vi "总氮总磷质控流程.vi"(0 "队列输入TP":refnum<queue>, 5 "总氮量程切换":enum32{"H", "L", "AUTO"}(ring)=enum."AUTO", 7 "总磷量程切换":enum32{"H", "L", "AUTO"}(ring)=enum."AUTO", 9 "总磷":bool, 11 "总氮":bool) -> (4 "布尔":bool, 6 "总磷中断报警":bool, 8 "总氮中断报警":bool)   [LabVIEW 2016, in "质控单元.lvlib"]
panel:
  out "总磷":bool
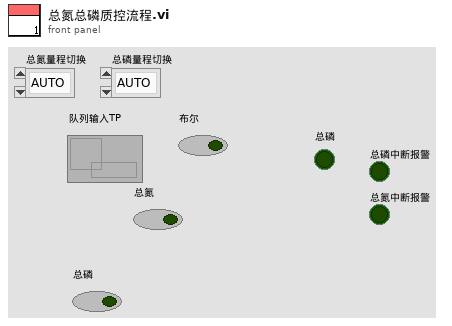
[diagram p1: front panel]
types:
  T1 = enum16{"待机", "启动氨氮水样", "氨氮测量中", "启动氨氮加标", "启动氨氮加标回收", "氨氮加标回收测量中", "启动总氮水样", "总氮测量中", "启动总氮加标", "启动总氮加标回收", "总氮加标回收测量中", "启动总磷水样", "总磷水样测量中", "启动总磷加标", "启动总磷加标回收", "总磷加标回收测量中", "结束"}
  T2 = cluster{"站号":u16, "量程切换":enum32{"H", "L", "AUTO"}, "控制命令":enum16{"启动测量", "标样核查", "零点核查", "跨度核查", "空白测试", "平行样测试", "加标回收", "空白校准", "标样校准", "初始化（清洗）", "停止测试", "仪器重启", "校时", "模式设置", "测量间隔设置"}, "模式设置":enum16{"待机", "连续模式", "周期模式", "定点模式", "受控模式", "手动模式"}, "测量间隔":u16}
  T3 = cluster{"时间标识":timestamp, "设备":string, "日志信息":string}
  T4 = cluster{"系统时间":timestamp, "工作状态":enum16{"空闲", "水样测试", "标样核查", "零点核查", "跨度核查", "空白测试", "平行样测试", "加标回收", "空白校准", "标样校准", "初始化（清洗）"}, "测量模式":enum16{"待机", "连续模式", "周期模式", "定点模式", "受控模式", "手动模式"}, "告警代码":enum16{"无告警", "缺试剂告警", "缺水样告警", "缺蒸馏水告警", "缺标液告警", "仪表漏液告警", "标定异常告警", "超量程告警", "加热异常", "低试剂预警", "超上限告警", "超下限告警", "仪表内部其他异常", "滴定异常告警", "电极异常告警", "量程切换告警", "参数设置告警", "PH电极电位异常", "电导率电极异常", "浊度光度异常", "溶解氧电极异常", "溶解氧光强异常", "温度异常告警", "PH异常告警", "溶解氧异常告警", "电导率异常告警", "浊度异常告警", "叶绿素异常告警", "藻密度异常告警", "蓝绿藻异常告警", "ORP异常告警", "氨氮异常告警", "清洁刷异常告警", "SD卡异常告警", "蓝牙异常告警", "Wifi异常告警", "流程异常告警"}, "故障代码":enum16{"无故障", "电机故障", "温度故障", "通讯故障", "滴定故障"}, "日志代码":u16, "软件版本":u16, "F0":sgl, "F1":sgl, "F2":sgl, "F3":sgl, "T":sgl, "H":sgl, "id":u16, "flowid":u16, "量程":u16, "总磷控温温度1":sgl, "营养盐控温温度2":sgl, "ADC":sgl}
  T5 = enum16{"空闲", "水样测试", "标样核查", "零点核查", "跨度核查", "空白测试", "平行样测试", "加标回收", "空白校准", "标样校准", "初始化（清洗）"}
  T6 = cluster{"因子编码":u32, "单位":u16, "标样参考值":sgl, "水样数据时间":timestamp, "水样实测值":sgl, "水样数据标识":string, "标样数据时间":timestamp, "标样实测值":sgl, "标样数据标识":string, "空白数据时间":timestamp, "空白实测值":sgl, "空白数据标识":string, "零点核查数据时间":timestamp, "零点核查实测值":sgl, "零点核查数据标识":string, "跨度核查数据时间":timestamp, "跨度核查实测值":sgl, "跨度核查数据标识":string, "加标回收数据时间":timestamp, "加标回收实测值":sgl, "加标回收数据标识":string, "平行样数据时间":timestamp, "平行样实测值":sgl, "平行样数据标识":string}
  T7 = cluster{"量程":dbl, "检出限":dbl, "加标前水样浓度":dbl, "加标后水样浓度":dbl, "加标水杯定容体积":dbl, "加标母液浓度":dbl, "加标体积":dbl, "加标回收率":dbl}
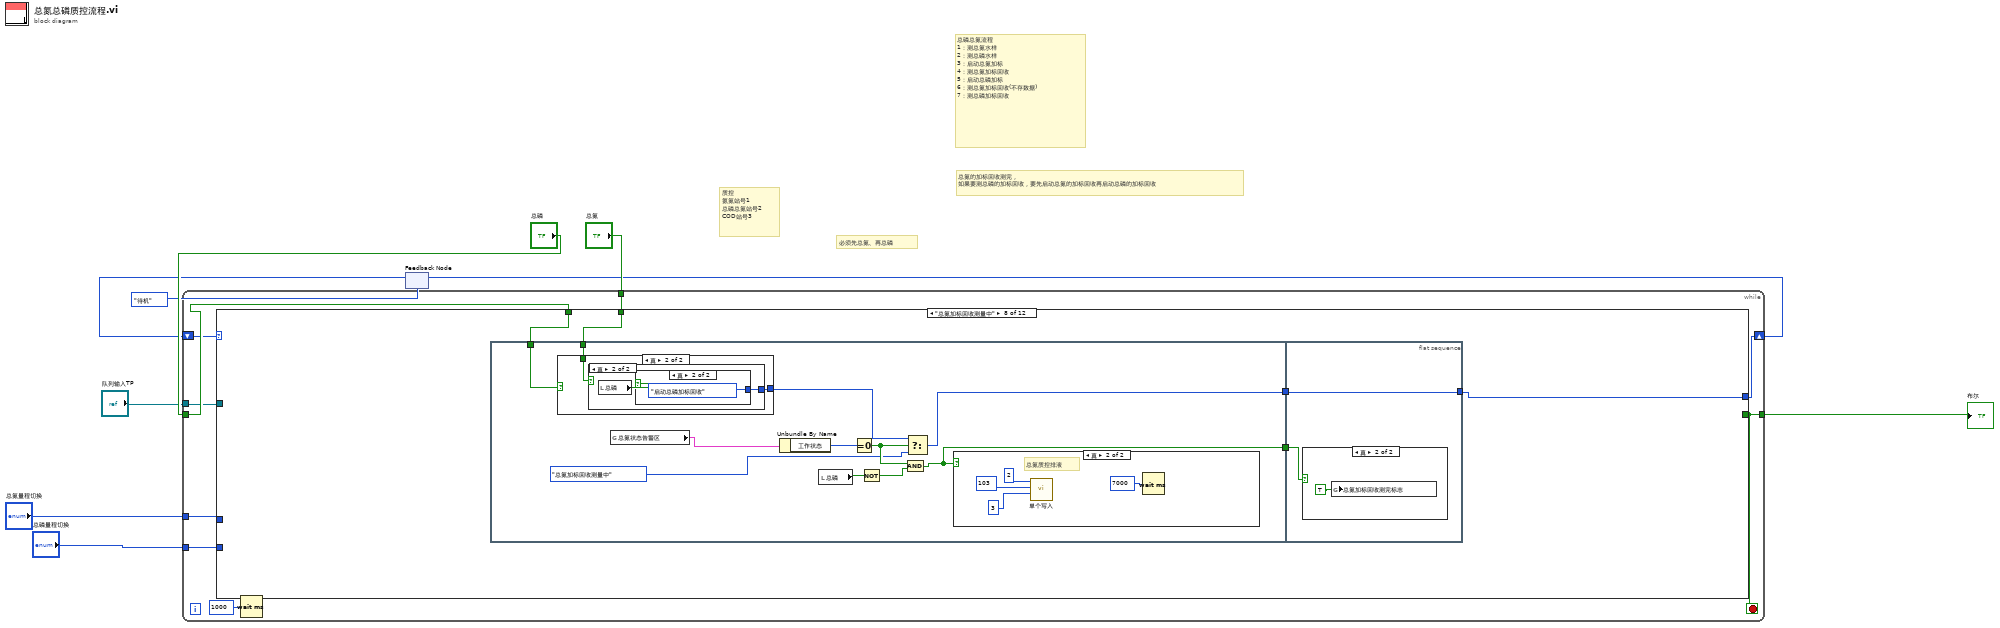
[diagram p0: block diagram]
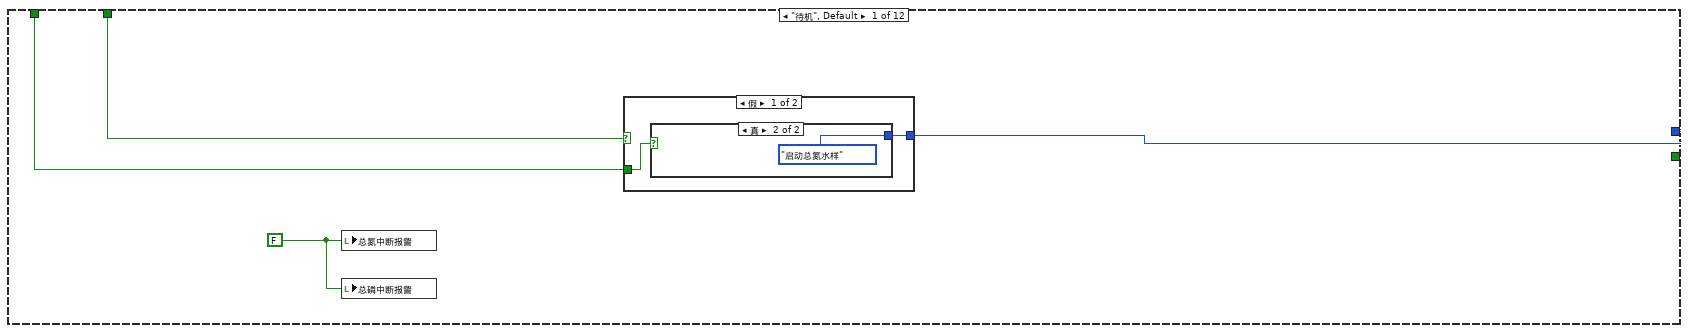
[diagram p2: hidden frame]
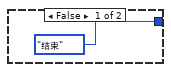
[diagram p3: hidden frame]
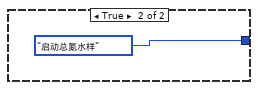
[diagram p4: hidden frame]
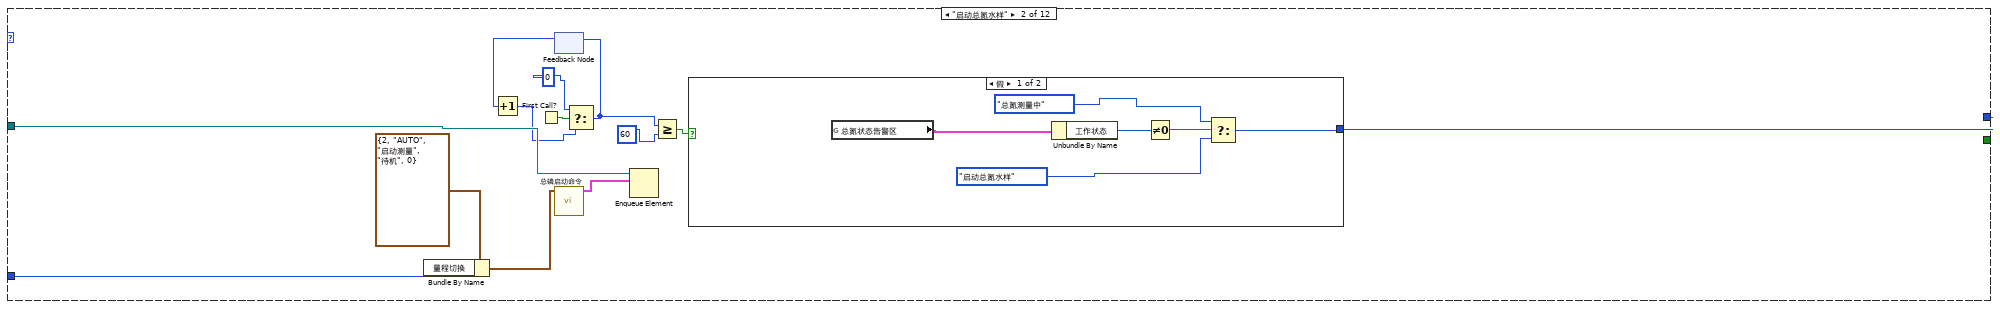
[diagram p5: hidden frame]
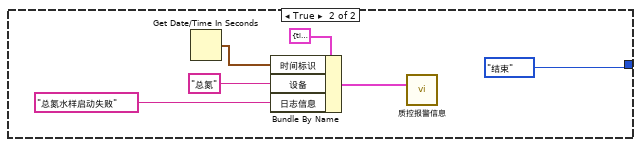
[diagram p6: hidden frame]
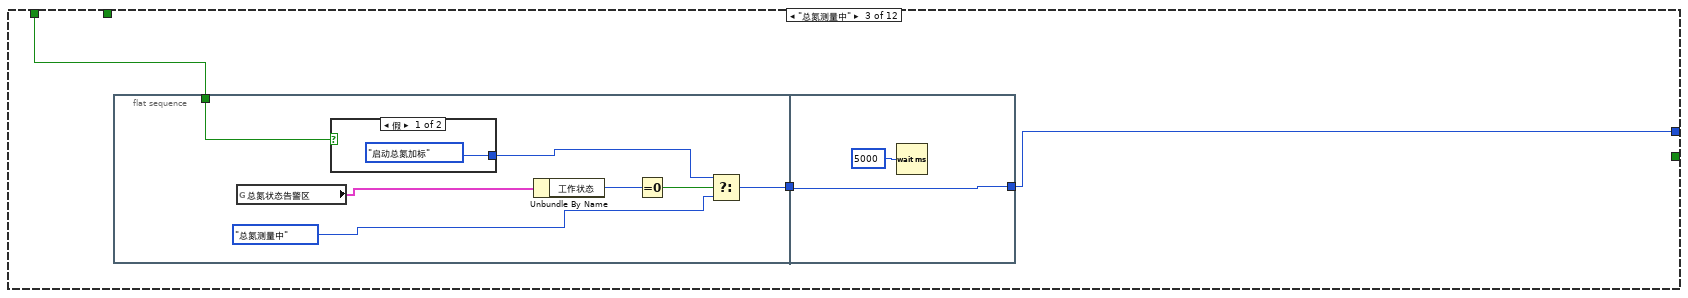
[diagram p7: hidden frame]
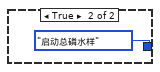
[diagram p8: hidden frame]
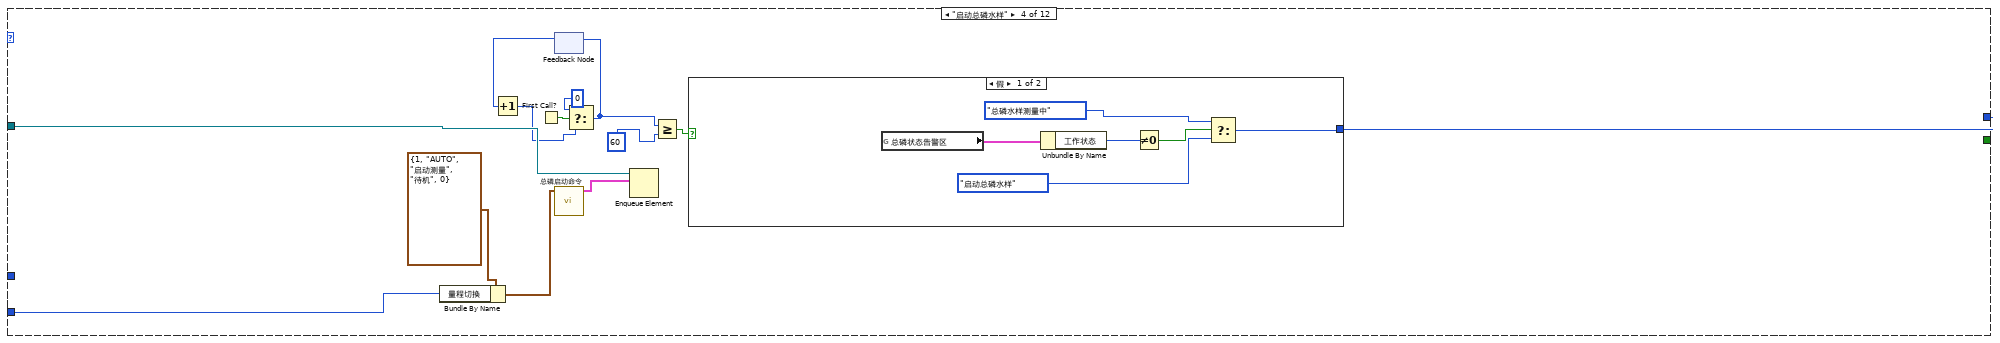
[diagram p9: hidden frame]
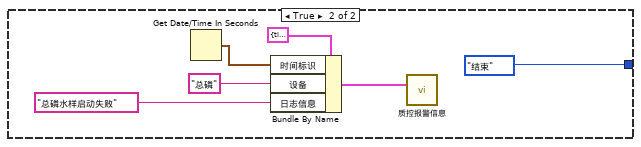
[diagram p10: hidden frame]
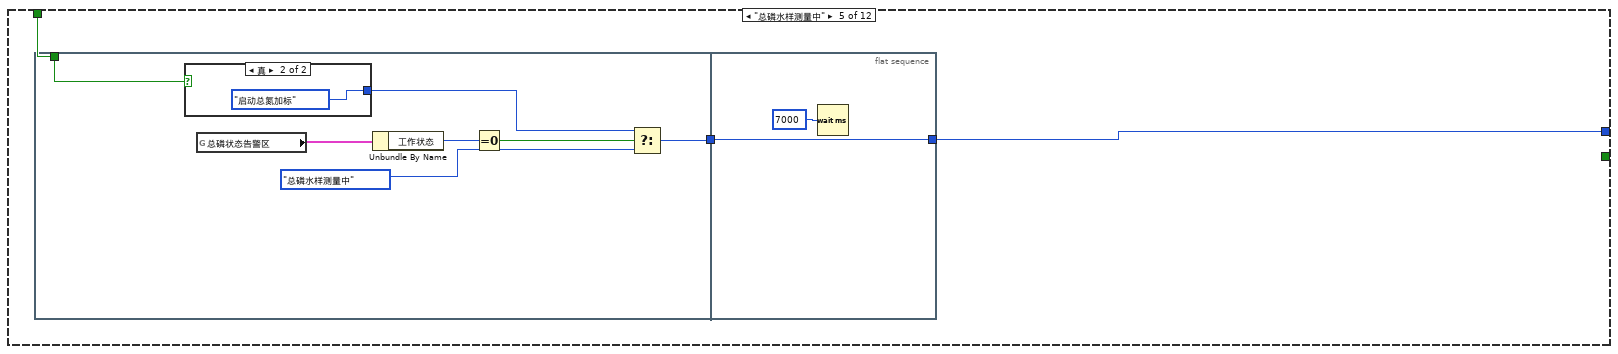
[diagram p11: hidden frame]
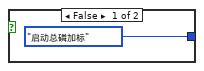
[diagram p12: hidden frame]
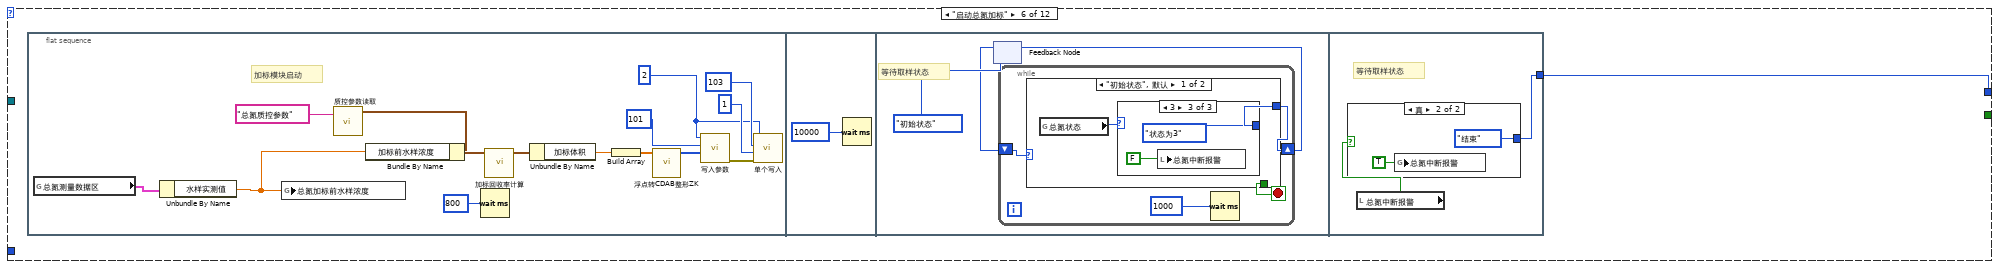
[diagram p13: hidden frame]
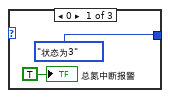
[diagram p14: hidden frame]
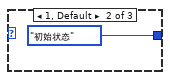
[diagram p15: hidden frame]
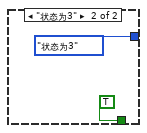
[diagram p16: hidden frame]
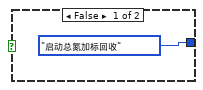
[diagram p17: hidden frame]
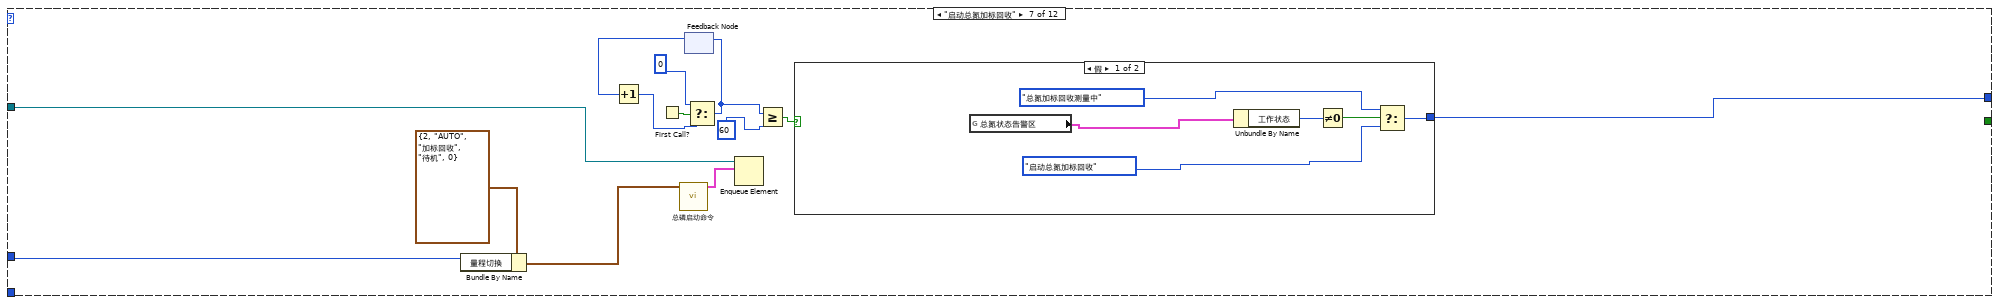
[diagram p18: hidden frame]
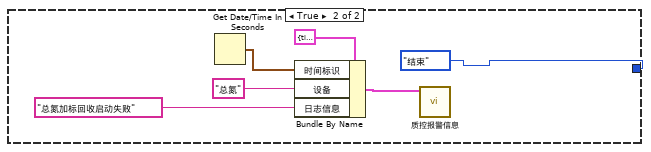
[diagram p19: hidden frame]
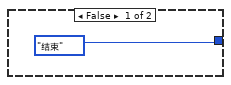
[diagram p20: hidden frame]
diagram:
  # "总磷总氮流程\n1：测总氮水样\n2：测总磷水样\n3：启动总氮加标\n4：测总氮加标回收\n5：启动总磷加标\n6：测总氮加标回收(不存数据)\n7：测总磷加标回收"
  # "总氮的加标回收测完，\n如果要测总磷的加标回收，要先启动总氮的加标回收再启动总磷的加标回收"
  # "质控\n氨氮站号1   \n总磷总氮站号2\nCOD站号3"
  # "必须先总氮、再总磷"
  n1 = feedback #1(T1."待机") -> (w1:T1)
  n2 = while {
    tunnel: "队列输入TP" -> [w17]
    tunnel: "总氮" -> [w16]
    tunnel: "总氮量程切换" -> [w14]
    tunnel: "总磷量程切换" -> [w13]
    shift-right: [w15] -> w4
    shift-left: w1 -> [w11]
    tunnel: "总磷" -> [w18]
    tunnel: [w12] -> w8
    stop <- w12 stop-if-true
    n3 = case shown="\"总氮加标回收测量中\"" w11 {
      tunnel: [w22 w39 w54 w78 w94 w106 w147 w171 w200 w244 w267 T1."结束"] -> w15
      tunnel: w17 -> [_ w40 _ w79 _ _ w149 _ _ w245 _ _]
      tunnel: [_ _ _ _ _ _ _ _ _ _ _ TRUE] -> w12
      tunnel: w18 -> [w21 _ w53 _ _ _ _ w172 _ _ _ _]
      tunnel: w16 -> [w20 _ _ _ w92 _ _ w170 _ _ _ _]
      tunnel: w14 -> [_ w28 _ _ _ _ w144 _ _ _ _ _]
      tunnel: w13 -> [_ _ _ w67 _ _ _ _ _ w240 _ _]
      frame "待机", Default {
        w19 = FALSE ("总氮中断报警")
        n4 = local write "总氮中断报警"(w19) -> ()
        n5 = local write "总磷中断报警"(w19) -> ()
        n6 = case shown="假" w20 {
          tunnel: w21 -> [w23 _]
          tunnel: [w24 T1."启动总氮水样"] -> w22
          frame False {
            n7 = case shown="真" w23 {
              tunnel: [T1."结束" T1."启动总氮水样"] -> w24
              frame False {
              }
              frame True {
              }
            }
          }
          frame True {
          }
        }
      }
      frame "启动总氮水样" {
        n8 = Bundle By Name(cluster=T2 {"站号"=2, "量程切换"=enum."AUTO", "控制命令"=enum."启动测量", "模式设置"=enum."待机", "测量间隔"=0} ("参数"), "量程切换"=w28) -> (w29:T2)
        n9 = First Call?() -> (First Call?: T/F=w37:bool)
        n10 = feedback #2() -> (w36:i32)  [unwired: 1 in]
        n11 = Increment(x=w36) -> (x+1=w35:i32)
        n12 = call "总磷启动命令.vi"("参数"=w29) -> ("启动命令"=w31:cluster{"命令":string, "data":variant})  [unwired: 10 in]
        n13 = Select(t=0, s=w37, f=w35) -> (s? t:f=w34:i32)
        n14 = feedback-in #2(w34) -> ()
        n15 = Enqueue Element(queue=w40, element=w31) -> ()  [unwired: 2 in, 3 out]
        n16 = Greater Or Equal?(x=w34, y=60) -> (x >= y?=w32:bool)
        n17 = case shown="假" w32 {
          tunnel: [w44 T1."结束"] -> w39
          frame False {
            n18 = global read "与总氮交互全局.vi" "总氮状态告警区"() -> (w41:T4)
            n19 = Unbundle By Name(w41) -> ("工作状态"=w45:T5)
            n20 = Not Equal To 0?(x=w45) -> (x != 0?=w46:bool)
            n21 = Select(t=T1."总氮测量中", s=w46, f=T1."启动总氮水样") -> (s? t:f=w44:T1)
          }
          frame True {
            n22 = Get Date/Time In Seconds() -> (seconds since 1Jan1904=w52:timestamp)
            n23 = Bundle By Name(cluster=T3 {"时间标识"=timestamp(0 s since 1904-01-01), "设备"="", "日志信息"=""} ("data in"), "时间标识"=w52, "设备"="总氮", "日志信息"="总氮水样启动失败") -> (w48:T3)
            n24 = call "质控报警信息.vi"("data in"=w48) -> ()  [unwired: 11 in]
          }
        }
      }
      frame "总氮测量中" {
        n25 = flat-sequence {
          tunnel: [w61] -> w55
          tunnel: w53 -> [w57]
          tunnel: [w66] -> w54
          tunnel: w55 -> [w66]
          frame #0 {
            n26 = global read "与总氮交互全局.vi" "总氮状态告警区"() -> (w56:T4)
            n27 = case shown="假" w57 {
              tunnel: [T1."启动总氮加标" T1."启动总磷水样"] -> w59
              frame False {
              }
              frame True {
              }
            }
            n28 = Unbundle By Name(w56) -> ("工作状态"=w62:T5)
            n29 = Equal To 0?(x=w62) -> (x = 0?=w60:bool)
            n30 = Select(t=w59, s=w60, f=T1."总氮测量中") -> (s? t:f=w61:T1)
          }
          frame #1 {
            n31 = Wait (ms)(milliseconds to wait=u32 5000 ("等待时间（毫秒）")) -> ()  [unwired: 1 out]
          }
        }
      }
      frame "启动总磷水样" {
        n32 = Bundle By Name(cluster=T2 {"站号"=1, "量程切换"=enum."AUTO", "控制命令"=enum."启动测量", "模式设置"=enum."待机", "测量间隔"=0} ("参数"), "量程切换"=w67) -> (w68:T2)
        n33 = First Call?() -> (First Call?: T/F=w76:bool)
        n34 = feedback #3() -> (w75:i32)  [unwired: 1 in]
        n35 = Increment(x=w75) -> (x+1=w74:i32)
        n36 = call "总磷启动命令.vi"("参数"=w68) -> ("启动命令"=w70:cluster{"命令":string, "data":variant})  [unwired: 10 in]
        n37 = Select(t=0, s=w76, f=w74) -> (s? t:f=w73:i32)
        n38 = feedback-in #3(w73) -> ()
        n39 = Enqueue Element(queue=w79, element=w70) -> ()  [unwired: 2 in, 3 out]
        n40 = Greater Or Equal?(x=w73, y=60) -> (x >= y?=w71:bool)
        n41 = case shown="假" w71 {
          tunnel: [w82 T1."结束"] -> w78
          frame False {
            n42 = global read "与总磷交互全局.vi" "总磷状态告警区"() -> (w83:T4)
            n43 = Unbundle By Name(w83) -> ("工作状态"=w84:T5)
            n44 = Not Equal To 0?(x=w84) -> (x != 0?=w85:bool)
            n45 = Select(t=T1."总磷水样测量中", s=w85, f=T1."启动总磷水样") -> (s? t:f=w82:T1)
          }
          frame True {
            n46 = Get Date/Time In Seconds() -> (seconds since 1Jan1904=w91:timestamp)
            n47 = Bundle By Name(cluster=T3 {"时间标识"=timestamp(0 s since 1904-01-01), "设备"="", "日志信息"=""} ("data in"), "时间标识"=w91, "设备"="总磷", "日志信息"="总磷水样启动失败") -> (w87:T3)
            n48 = call "质控报警信息.vi"("data in"=w87) -> ()  [unwired: 11 in]
          }
        }
      }
      frame "总磷水样测量中" {
        n49 = flat-sequence {
          tunnel: [w99] -> w93
          tunnel: w92 -> [w96]
          tunnel: [w105] -> w94
          tunnel: w93 -> [w105]
          frame #0 {
            n50 = case shown="真" w96 {
              tunnel: [T1."启动总磷加标" T1."启动总氮加标"] -> w97
              frame False {
              }
              frame True {
              }
            }
            n51 = global read "与总磷交互全局.vi" "总磷状态告警区"() -> (w100:T4)
            n52 = Unbundle By Name(w100) -> ("工作状态"=w101:T5)
            n53 = Equal To 0?(x=w101) -> (x = 0?=w98:bool)
            n54 = Select(t=w97, s=w98, f=T1."总磷水样测量中") -> (s? t:f=w99:T1)
          }
          frame #1 {
            n55 = Wait (ms)(milliseconds to wait=u32 7000 ("等待时间（毫秒）")) -> ()  [unwired: 1 out]
          }
        }
      }
      frame "启动总氮加标" {
        n56 = flat-sequence {
          tunnel: [w140] -> w106
          frame #0 {
            w108 = u16 2 ("value")
            # "加标模块启动"
            n57 = global read "与总氮交互全局.vi" "总氮测量数据区"() -> (w107:T6)
            n58 = Unbundle By Name(w107) -> ("水样实测值"=w109:sgl)
            n59 = global write "水样浓度全局.vi" "总氮加标前水样浓度"(w109) -> ()
            n60 = call "质控参数读取.vi"("section"="总氮质控参数") -> ("参数"=w111:T7)  [unwired: 9 in, 1 out]
            n61 = Bundle By Name(cluster=w111, "加标前水样浓度"=w109) -> (w120:T7)
            n62 = Wait (ms)(milliseconds to wait=u32 800 ("等待时间（毫秒）")) -> ()  [unwired: 1 out]
            n63 = call "加标回收率计算.vi"("参数"=w120) -> ("参数 out"=w119:T7)  [unwired: 10 in]
            n64 = Unbundle By Name(w119) -> ("加标体积"=w112:dbl)
            n65 = Build Array(w112) -> (w118:dbl[])
            n66 = call "浮点转CDAB整形ZK.vi"("浮点数"=w118) -> ("CDAB整形输出"=w113:u16[])  [unwired: 10 in]
            n67 = call "写入参数.vi"("values"=w113, "starting address"=u16 101, "Slave ID"=w108) -> ("error out"=w117:errorcluster)  [unwired: 8 in]
            n68 = call "单个写入.vi"("Error in"=w117, "value"=u16 1, "address"=u16 103, "Slave ID"=w108) -> ()  [unwired: 7 in, 1 out]
          }
          frame #1 {
            n69 = Wait (ms)(milliseconds to wait=u32 10000 ("等待时间（毫秒）")) -> ()  [unwired: 1 out]
          }
          frame #2 {
            # "等待取样状态"
            n70 = feedback #4(enum16{"初始状态", "状态为3"}."初始状态") -> (w124:enum16{"初始状态", "状态为3"})
            n71 = while {
              shift-right: [w128] -> w123
              shift-left: w124 -> [w129]
              stop <- w127 stop-if-true
              n72 = case shown="\"初始状态\", 默认" w129 {
                tunnel: [w131 enum16{"初始状态", "状态为3"}."状态为3"] -> w128
                tunnel: [_ TRUE] -> w127
                frame "初始状态", Default {
                  n73 = global read "加标回收状态全局变量.vi" "总氮状态"() -> (w130:u16)
                  n74 = case shown="3" w130 {
                    tunnel: [enum16{"初始状态", "状态为3"}."状态为3" enum16{"初始状态", "状态为3"}."初始状态" enum16{"初始状态", "状态为3"}."状态为3"] -> w131
                    frame 0 {
                      "总氮中断报警" <- TRUE ("总氮中断报警")
                    }
                    frame 1, Default {
                    }
                    frame 3 {
                      n75 = local write "总氮中断报警"(FALSE ("总氮中断报警")) -> ()
                    }
                  }
                }
                frame "状态为3" {
                }
              }
              n76 = Wait (ms)(milliseconds to wait=u32 1000 ("等待时间（毫秒）")) -> ()  [unwired: 1 out]
            }
            n77 = feedback-in #4(w123) -> ()
          }
          frame #3 {
            # "等待取样状态"
            n78 = local read "总氮中断报警"() -> (w139:bool)
            n79 = case shown="真" w139 {
              tunnel: [T1."启动总氮加标回收" T1."结束"] -> w140
              frame False {
              }
              frame True {
                n80 = global write "质控中断报警全局.vi" "总氮中断报警"(TRUE ("总氮中断报警")) -> ()
              }
            }
          }
        }
      }
      frame "启动总氮加标回收" {
        n81 = Bundle By Name(cluster=T2 {"站号"=2, "量程切换"=enum."AUTO", "控制命令"=enum."加标回收", "模式设置"=enum."待机", "测量间隔"=0} ("参数"), "量程切换"=w144) -> (w145:T2)
        n82 = First Call?() -> (First Call?: T/F=w155:bool)
        n83 = call "总磷启动命令.vi"("参数"=w145) -> ("启动命令"=w148:cluster{"命令":string, "data":variant})  [unwired: 10 in]
        n84 = feedback #5() -> (w154:i32)  [unwired: 1 in]
        n85 = Increment(x=w154) -> (x+1=w153:i32)
        n86 = Select(t=0, s=w155, f=w153) -> (s? t:f=w152:i32)
        n87 = feedback-in #5(w152) -> ()
        n88 = Enqueue Element(queue=w149, element=w148) -> ()  [unwired: 2 in, 3 out]
        n89 = Greater Or Equal?(x=w152, y=60) -> (x >= y?=w150:bool)
        n90 = case shown="假" w150 {
          tunnel: [w160 T1."结束"] -> w147
          frame False {
            n91 = global read "与总氮交互全局.vi" "总氮状态告警区"() -> (w157:T4)
            n92 = Unbundle By Name(w157) -> ("工作状态"=w162:T5)
            n93 = Not Equal To 0?(x=w162) -> (x != 0?=w161:bool)
            n94 = Select(t=T1."总氮加标回收测量中", s=w161, f=T1."启动总氮加标回收") -> (s? t:f=w160:T1)
          }
          frame True {
            n95 = Get Date/Time In Seconds() -> (seconds since 1Jan1904=w168:timestamp)
            n96 = Bundle By Name(cluster=T3 {"时间标识"=timestamp(0 s since 1904-01-01), "设备"="", "日志信息"=""} ("data in"), "时间标识"=w168, "设备"="总氮", "日志信息"="总氮加标回收启动失败") -> (w164:T3)
            n97 = call "质控报警信息.vi"("data in"=w164) -> ()  [unwired: 11 in]
          }
        }
      }
      frame "总氮加标回收测量中" {
        n98 = flat-sequence {
          tunnel: [w183] -> w173
          tunnel: w172 -> [w180]
          tunnel: w170 -> [w176]
          tunnel: [w174] -> w169
          tunnel: [w198] -> w171
          tunnel: w173 -> [w198]
          tunnel: w169 -> [w197]
          frame #0 {
            n99 = case shown="真" w180 {
              tunnel: [T1."结束" w187] -> w182
              tunnel: w176 -> [_ w186]
              frame False {
              }
              frame True {
                n100 = case shown="真" w186 {
                  tunnel: [T1."启动总磷加标回收" w190] -> w187
                  frame False {
                  }
                  frame True {
                    n101 = local read "总磷"() -> (w189:bool)
                    n102 = case shown="真" w189 {
                      tunnel: [T1."启动总磷加标" T1."启动总磷加标回收"] -> w190
                      frame False {
                      }
                      frame True {
                      }
                    }
                  }
                }
              }
            }
            n103 = global read "与总氮交互全局.vi" "总氮状态告警区"() -> (w175:T4)
            n104 = Unbundle By Name(w175) -> ("工作状态"=w184:T5)
            n105 = local read "总磷"() -> (w178:bool)
            n106 = Equal To 0?(x=w184) -> (x = 0?=w181:bool)
            n107 = Not(x=w178) -> (.not. x?=w177:bool)
            n108 = And(x=w181, y=w177) -> (x .and. y?=w174:bool)
            n109 = Select(t=w182, s=w181, f=T1."总氮加标回收测量中") -> (s? t:f=w183:T1)
            n110 = case shown="真" w174 {
              frame False {
              }
              frame True {
                # "总氮质控排液"
                n111 = call "单个写入.vi"("value"=u16 3, "address"=u16 103, "Slave ID"=u8 2) -> ()  [unwired: 8 in, 1 out]
                n112 = Wait (ms)(milliseconds to wait=u32 7000 ("等待时间（毫秒）")) -> ()  [unwired: 1 out]
              }
            }
          }
          frame #1 {
            n113 = case shown="真" w197 {
              frame False {
              }
              frame True {
                n114 = global write "质控测完标志全局 1.vi" "总氮加标回收测完标志"(TRUE) -> ()
              }
            }
          }
        }
      }
      frame "启动总磷加标" {
        n115 = flat-sequence {
          tunnel: [w236] -> w200
          frame #0 {
            n116 = Wait (ms)(milliseconds to wait=u32 180000 ("等待时间（毫秒）")) -> ()  [unwired: 1 out]
          }
          frame #1 {
            w207 = u16 2 ("value")
            # "加标模块启动"
            n117 = global read "与总磷交互全局.vi" "总磷测量数据区"() -> (w203:T6)
            n118 = Unbundle By Name(w203) -> ("水样实测值"=w202:sgl)
            n119 = call "质控参数读取.vi"("section"="总磷质控参数") -> ("参数"=w205:T7)  [unwired: 9 in, 1 out]
            n120 = Bundle By Name(cluster=w205, "加标前水样浓度"=w202) -> (w215:T7)
            n121 = global write "水样浓度全局.vi" "总磷加标前水样浓度"(w202) -> ()
            n122 = Wait (ms)(milliseconds to wait=u32 800 ("等待时间（毫秒）")) -> ()  [unwired: 1 out]
            n123 = call "加标回收率计算.vi"("参数"=w215) -> ("参数 out"=w214:T7)  [unwired: 10 in]
            n124 = Unbundle By Name(w214) -> ("加标体积"=w206:dbl)
            n125 = Build Array(w206) -> (w213:dbl[])
            n126 = call "浮点转CDAB整形ZK.vi"("浮点数"=w213) -> ("CDAB整形输出"=w208:u16[])  [unwired: 10 in]
            n127 = call "写入参数.vi"("values"=w208, "starting address"=u16 101, "Slave ID"=w207) -> ("error out"=w212:errorcluster)  [unwired: 8 in]
            n128 = call "单个写入.vi"("Error in"=w212, "value"=u16 1, "address"=u16 103, "Slave ID"=w207) -> ()  [unwired: 7 in, 1 out]
          }
          frame #2 {
            n129 = Wait (ms)(milliseconds to wait=u32 10000 ("等待时间（毫秒）")) -> ()  [unwired: 1 out]
          }
          frame #3 {
            # "等待取样状态"
            n130 = feedback #6(enum16{"初始状态", "状态为3"}."初始状态") -> (w219:enum16{"初始状态", "状态为3"})
            n131 = while {
              shift-right: [w223] -> w218
              shift-left: w219 -> [w224]
              stop <- w222 stop-if-true
              n132 = case shown="\"状态为3\"" w224 {
                tunnel: [w226 enum16{"初始状态", "状态为3"}."状态为3"] -> w223
                tunnel: [_ TRUE] -> w222
                frame "初始状态", Default {
                  n133 = global read "加标回收状态全局变量.vi" "总磷状态"() -> (w225:u16)
                  n134 = case shown="0" w225 {
                    tunnel: [enum16{"初始状态", "状态为3"}."状态为3" enum16{"初始状态", "状态为3"}."初始状态" enum16{"初始状态", "状态为3"}."状态为3"] -> w226
                    frame 0 {
                      "总磷中断报警" <- TRUE ("总磷中断报警")
                    }
                    frame 1, Default {
                    }
                    frame 3 {
                      n135 = local write "总磷中断报警"(FALSE ("总磷中断报警")) -> ()
                    }
                  }
                }
                frame "状态为3" {
                  "总磷" <- TRUE
                }
              }
              n136 = Wait (ms)(milliseconds to wait=u32 1000 ("等待时间（毫秒）")) -> ()  [unwired: 1 out]
            }
            n137 = feedback-in #6(w218) -> ()
          }
          frame #4 {
            n138 = local read "总磷中断报警"() -> (w235:bool)
            n139 = case shown="真" w235 {
              tunnel: [T1."启动总氮加标回收" T1."结束"] -> w236
              frame False {
                # "等待取样状态"
              }
              frame True {
                n140 = global write "质控中断报警全局.vi" "总磷中断报警"(TRUE ("总磷中断报警")) -> ()
              }
            }
          }
        }
      }
      frame "启动总磷加标回收" {
        n141 = Bundle By Name(cluster=T2 {"站号"=1, "量程切换"=enum."AUTO", "控制命令"=enum."加标回收", "模式设置"=enum."待机", "测量间隔"=0} ("参数"), "量程切换"=w240) -> (w241:T2)
        n142 = First Call?() -> (First Call?: T/F=w252:bool)
        n143 = feedback #7() -> (w251:i32)  [unwired: 1 in]
        n144 = Increment(x=w251) -> (x+1=w250:i32)
        n145 = call "总磷启动命令.vi"("参数"=w241) -> ("启动命令"=w246:cluster{"命令":string, "data":variant})  [unwired: 10 in]
        n146 = Select(t=0, s=w252, f=w250) -> (s? t:f=w249:i32)
        n147 = feedback-in #7(w249) -> ()
        n148 = Enqueue Element(queue=w245, element=w246) -> ()  [unwired: 2 in, 3 out]
        n149 = Greater Or Equal?(x=w249, y=60) -> (x >= y?=w247:bool)
        n150 = case shown="真" w247 {
          tunnel: [w256 T1."结束"] -> w244
          frame False {
            n151 = global read "与总磷交互全局.vi" "总磷状态告警区"() -> (w257:T4)
            n152 = Unbundle By Name(w257) -> ("工作状态"=w258:T5)
            n153 = Not Equal To 0?(x=w258) -> (x != 0?=w259:bool)
            n154 = Select(t=T1."总磷加标回收测量中", s=w259, f=T1."启动总磷加标回收") -> (s? t:f=w256:T1)
          }
          frame True {
            n155 = Get Date/Time In Seconds() -> (seconds since 1Jan1904=w265:timestamp)
            n156 = Bundle By Name(cluster=T3 {"时间标识"=timestamp(0 s since 1904-01-01), "设备"="", "日志信息"=""} ("data in"), "时间标识"=w265, "设备"="总磷", "日志信息"="总磷加标回收启动失败") -> (w261:T3)
            n157 = call "质控报警信息.vi"("data in"=w261) -> ()  [unwired: 11 in]
          }
        }
        n158 = local write "总磷"(FALSE ("总磷")) -> ()
      }
      frame "总磷加标回收测量中" {
        n159 = flat-sequence {
          tunnel: [w272] -> w268
          tunnel: [w269] -> w266
          tunnel: [w280] -> w267
          tunnel: w268 -> [w280]
          tunnel: w266 -> [w279]
          frame #0 {
            n160 = global read "与总磷交互全局.vi" "总磷状态告警区"() -> (w273:T4)
            n161 = Unbundle By Name(w273) -> ("工作状态"=w274:T5)
            n162 = Equal To 0?(x=w274) -> (x = 0?=w269:bool)
            n163 = Select(t=T1."结束", s=w269, f=T1."总磷加标回收测量中") -> (s? t:f=w272:T1)
            n164 = case shown="真" w269 {
              frame False {
              }
              frame True {
                # "总磷质控排液"
                n165 = Wait (ms)(milliseconds to wait=u32 5000 ("等待时间（毫秒）")) -> ()  [unwired: 1 out]
                n166 = call "单个写入.vi"("value"=u16 3, "address"=u16 103, "Slave ID"=u8 2) -> ()  [unwired: 8 in, 1 out]
              }
            }
          }
          frame #1 {
            n167 = case shown="真" w279 {
              frame False {
              }
              frame True {
                n168 = global write "质控测完标志全局 1.vi" "总磷加标回收测完标志"(TRUE) -> ()
              }
            }
          }
        }
      }
      frame "结束" {
        n169 = Wait (ms)(milliseconds to wait=u32 5000 ("等待时间（毫秒）")) -> ()  [unwired: 1 out]
      }
    }
    n170 = Wait (ms)(milliseconds to wait=u32 1000 ("等待时间（毫秒）")) -> ()  [unwired: 1 out]
  }
  "布尔" <- w8
  n171 = feedback-in #1(w4) -> ()
